vi "SigMath Class - Set FP Position.vi"(5 "error in (no error)":errorcluster) -> (19 "error out":errorcluster)   [LabVIEW 2022 SP3, in "SigMath.lvclass"]
uses:
  SigMath.lvclass
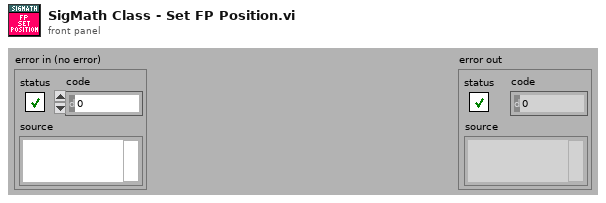
[diagram p1: front panel]
types:
  T1 = typedef "SigMath.lvclass/ClassAttributes.ctl" = cluster{"Window List":refnum<vi>[]}
  T2 = typedef "LVRectTypeDef.ctl" = cluster{"Left":i16, "Top":i16, "Right":i16, "Bottom":i16}
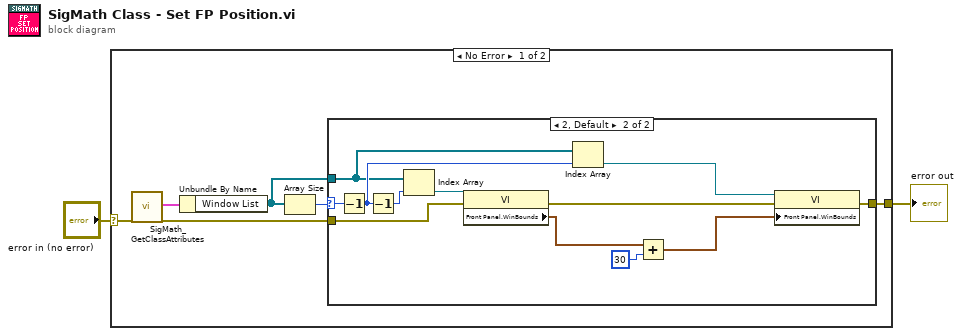
[diagram p0: block diagram]
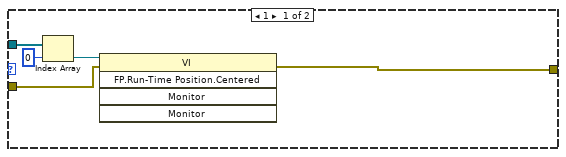
[diagram p2: hidden frame]
diagram:
  n1 = case shown="No Error" "error in (no error)" {
    selector: "error in (no error)" -> [w8 w26]
    tunnel: [w3 w26] -> w1
    frame No Error {
      n2 = call "SigMath_GetClassAttributes.vi"("error in (no error)"=w8) -> ("class attributes"=w7:T1, "error out"=w4:errorcluster)  [unwired: 15 in, 2 out]
      n3 = Unbundle By Name(w7) -> ("Window List"=w5:refnum<vi>[])
      n4 = Array Size(array=w5) -> (size(s)=w6:i32)
      n5 = case shown="2, Default" w6 {
        selector: w6 -> [_ w25]
        tunnel: w5 -> [w13 w20]
        tunnel: w4 -> [w10 w22]
        tunnel: [w9 w17] -> w3
        frame 1 {
          n6 = Index Array(array=w13, index=0) -> (element=w11:refnum<vi>)
          n7 = invoke class="VI" method="FP.Run-Time Position.Centered"(reference=w11, error in=w10) -> (error out=w9:errorcluster)  [unwired: 3 in, 4 out]
        }
        frame 2, Default {
          n8 = Decrement(x=w25) -> (x-1=w21:i32)
          n9 = Decrement(x=w21) -> (x-1=w24:i32)
          n10 = Index Array(array=w20, index=w24) -> (element=w23:refnum<vi>)
          n11 = property class="VI"(reference=w23, error in=w22) -> (error out=w19:errorcluster, "Front Panel.WinBounds"=w16:T2)  [unwired: 1 out]
          n12 = Index Array(array=w20, index=w21) -> (element=w18:refnum<vi>)
          n13 = Add(x=w16, y=i16 30 ("Right")) -> (x+y=w14:T2)
          n14 = property class="VI"(reference=w18, error in=w19, "Front Panel.WinBounds"=w14) -> (error out=w17:errorcluster)  [unwired: 1 out]
        }
      }
    }
    frame Error {
    }
  }
  "error out" <- w1
